vi "Delete Agent Refnum.vi"(8 "error in (no error)":errorcluster, 11 "agent":T2) -> (0 "error out":errorcluster, 3 "LIBSSH2_AGENT*":u64, 5 "session":T1)   [LabVIEW 2017, in "libssh2.lvlib"]
uses:
  libssh2.lvlib
  Agent Refnum.ctl
  Session Refnum.ctl
  Agent Refnum Data.ctl
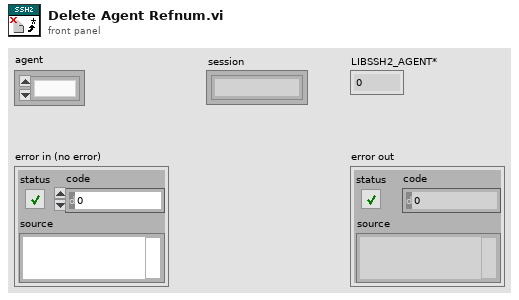
[diagram p1: front panel]
types:
  T1 = typedef "libssh2.lvlib/Session Refnum.ctl" = refnum<k1>
  T2 = typedef "libssh2.lvlib/Agent Refnum.ctl" = refnum<k1>
  T3 = typedef "libssh2.lvlib/Agent Refnum Data.ctl" = cluster{"LIBSSH2_AGENT*":u64, "session":T1}
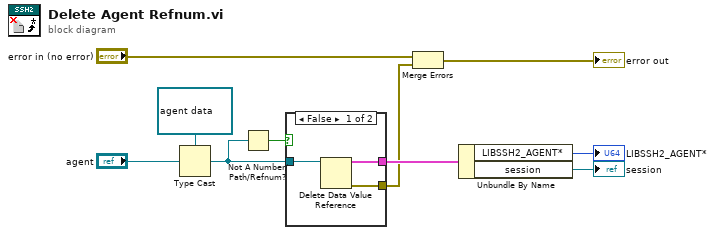
[diagram p0: block diagram]
diagram:
  n1 = Type Cast(type=refnum<data-value> refnum ("data value reference"), x="agent") -> (*(type *) &x=w6:refnum<data-value>)
  n2 = Not A Number/Path/Refnum?(number/path/refnum=w6) -> (NaN/Path/Refnum?=w5:bool)
  n3 = case shown="False" w5 {
    tunnel: [w13 _] -> w8
    tunnel: [w12 _] -> w7
    tunnel: w6 -> [w11 _]
    frame False {
      n4 = Delete Data Value Reference(data value reference=w11) -> (data value=w13:T3, error out=w12:errorcluster)  [unwired: 1 in]
    }
    frame True {
    }
  }
  n5 = Merge Errors("error in (no error)", w7) -> (→"error out":errorcluster)
  n6 = Unbundle By Name(w8) -> ("LIBSSH2_AGENT*"=→"LIBSSH2_AGENT*":u64, "session"=→"session":T1)
